vi "Load McP ScanArray.dat.V1.00.vi"(0 "McP Counter Position Path":path, 1 "WholeArray?":bool) -> (2 "ScanPattern":string, 3 "Position":sgl format="%.10e", 4 "EOF?":bool)   [LabVIEW 2025]
doc: "Author: Scott Hannahs <sth@magnet.fsu.edu>\n\nThis software is licensed for use under the “MIT License\"\nCopyright (c) 2025 Scott Hannahs, sth@sth@magnet.sthnet.net\n\nPermission is hereby granted, free of charge, to any person obtaining a copy of this software and associated documentation files (the \"Software\"), to deal in the Software without restriction, including without limitation the rights to use, copy, modify, merge, publish, distribute, sublicense, and/or sell copies of the Software, and to permit persons to whom the Software is furnished to do so, subject to the following conditions: The above copyright notice and this permission notice shall be included in all copies or substantial portions of the Software.\n\nTHE SOFTWARE IS PROVIDED \"AS IS\", WITHOUT WARRANTY OF ANY KIND, EXPRESS OR IMPLIED, INCLUDING BUT NOT LIMITED TO THE WARRANTIES OF MERCHANTABILITY, FITNESS FOR A PARTICULAR PURPOSE AND NONINFRINGEMENT. IN NO EVENT SHALL THE AUTHORS OR COPYRIGHT HOLDERS BE LIABLE FOR ANY CLAIM, DAMAGES OR OTHER LIABILITY, WHETHER IN AN ACTION OF CONTRACT, TORT OR OTHERWISE, ARISING FROM, OUT OF OR IN CONNECTION WITH THE SOFTWARE OR THE USE OR OTHER DEALINGS IN THE SOFTWARE."
uses:
  <vilib>/Utility/file.llb/Read From Spreadsheet File (DBL).vi
panel:
  in  "start of read offset (chars.:0 )":i32
  out "mark after read (chars.)":i32
  out "McP ScanArray.dat Path":path
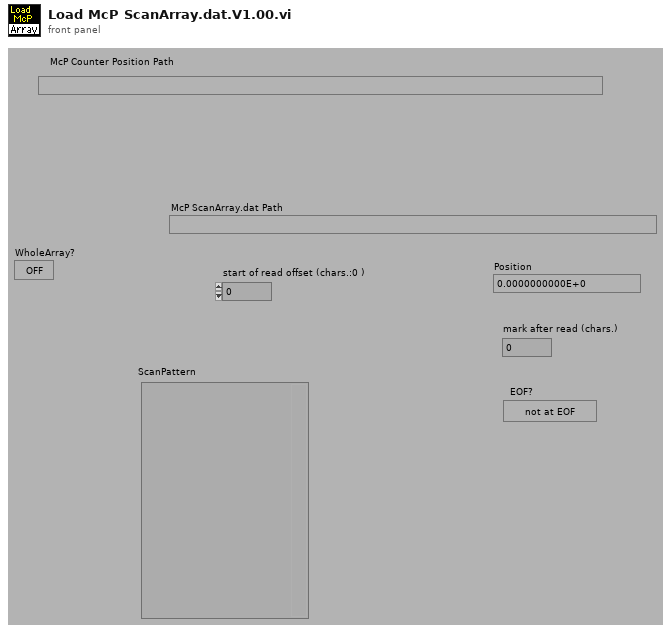
[diagram p1: front panel]
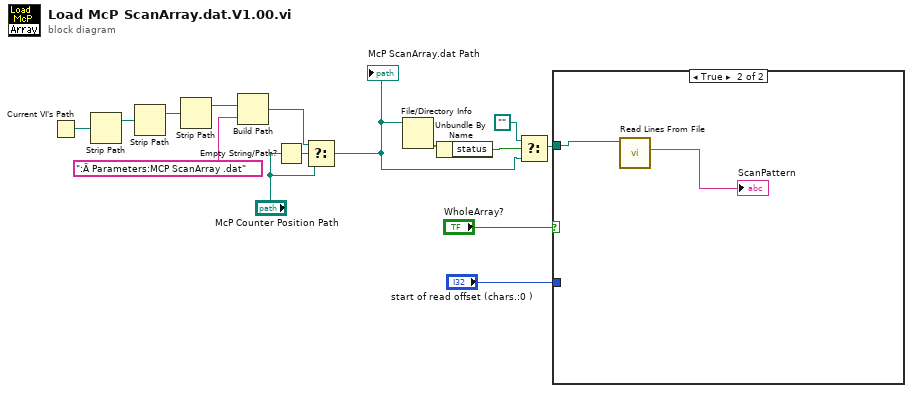
[diagram p0: block diagram]
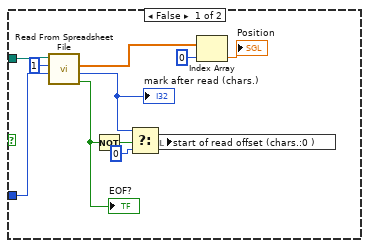
[diagram p2: hidden frame]
diagram:
  n1 = Current VI's Path() -> (path=w6:path)
  n2 = Strip Path(path=w6) -> (stripped path=w11:path)  [unwired: 1 out]
  n3 = Strip Path(path=w11) -> (stripped path=w10:path)  [unwired: 1 out]
  n4 = Strip Path(path=w10) -> (stripped path=w7:path)  [unwired: 1 out]
  n5 = Build Path(base path=w7, name or relative path=":Ä Parameters:MCP ScanArray .dat") -> (appended path=w5:path)
  n6 = Empty String/Path?(string/path="McP Counter Position Path") -> (empty?=w12:bool)
  n7 = Select(t=w5, s=w12, f="McP Counter Position Path") -> (s? t:f=w4:path)
  "McP ScanArray.dat Path" <- w4
  n8 = File/Directory Info(path=w4) -> (error out=w15:errorcluster)  [unwired: 1 in, 6 out]
  n9 = Unbundle By Name(w15) -> ("status"=w14:bool)
  n10 = Select(t=path "", s=w14, f=w4) -> (s? t:f=w3:path)
  n11 = case shown="True" "WholeArray?" {
    tunnel: w3 -> [w26 w28]
    tunnel: "start of read offset (chars.:0 )" -> [w25 _]
    frame False {
      n12 = call-poly <vilib>:"Read From Spreadsheet File.vi"("start of read offset (chars.:0)"=w25, "number of rows (all:-1)"=1, "file path (dialog if empty)"=w26) -> ("EOF?"=w23:bool, "mark after read (chars.)"=w21:i32, "first row"=w16:dbl[])  [unwired: 4 in, 2 out]
      "mark after read (chars.)" <- w21
      "EOF?" <- w23
      n13 = Not(x=w23) -> (.not. x?=w22:bool)
      n14 = Select(t=w21, s=w22, f=0) -> (s? t:f=w20:i32)
      n15 = local write "start of read offset (chars.:0 )"(w20) -> ()
      n16 = Index Array(array=w16, index=0 ("Index")) -> (element=→"Position":dbl)
    }
    frame True {
      n17 = call <vilib>:"Read Lines From File.vi"("file path (dialog if empty)"=w28) -> ("line string"=→"ScanPattern":string)  [unwired: 5 in, 3 out]
    }
  }
